vi "Write Behavior.vi"(10 "Behavior":T1(ring)=enum."Default", 11 "Philips Dialog in":refnum<class "Flex UI Dialog.lvclass">) -> (3 "Philips Dialog out":refnum<class "Flex UI Dialog.lvclass">)   [LabVIEW 2014, in "Flex UI Dialog.lvclass"]
uses:
  Flex UI Dialog.lvclass
  Flex UI Dialog.lvclass/Flex UI Dialog.ctl
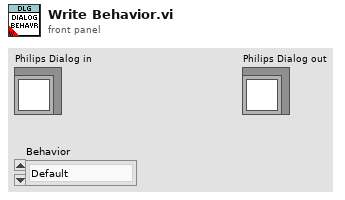
[diagram p1: front panel]
types:
  T1 = enum32{"Invalid", "Default", "Floating", "Floating/Auto-Hide", "Modal"}
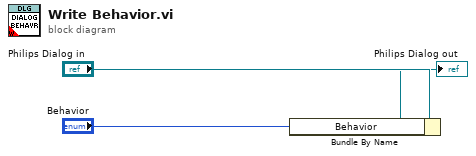
[diagram p0: block diagram]
diagram:
  n1 = Bundle By Name(cluster="Philips Dialog in", "Behavior"="Behavior") -> (→"Philips Dialog out":refnum<class "Flex UI Dialog.lvclass">)
